vi "ABB SIgn All.vi"(11 "ImageFolder":path) -> ()   [LabVIEW 2017]
uses:
  ABB global.vi
panel:
  out "Signatures":T1(array[cluster])
  out "Please Sign":string
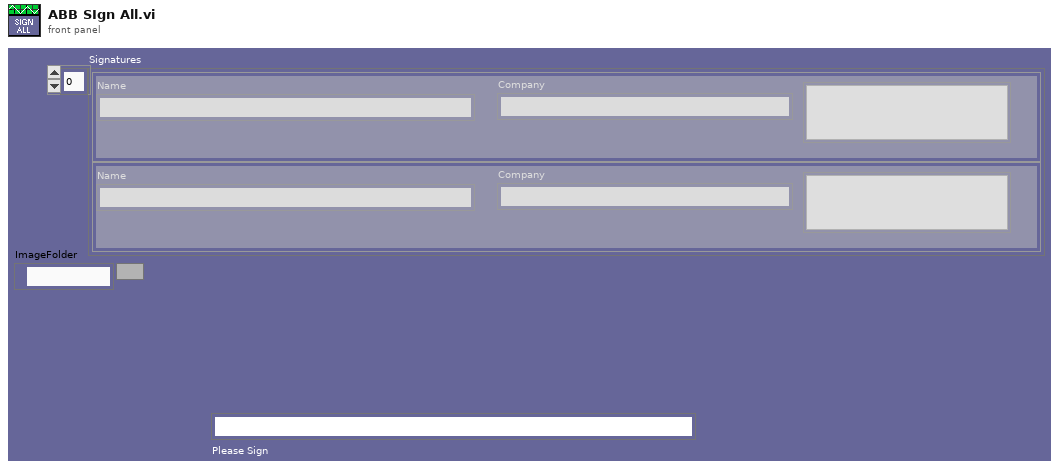
[diagram p1: front panel]
types:
  T1 = cluster{"Name":string, "Company":string, "new picture":picture}[]
  T2 = cluster{"String":string, "String":string, "new picture":picture}[]
  T3 = cluster{"String":string, "String":string, "Signature":picture}
  T4 = cluster{"String":string, "String":string, "Signature":picture}[]
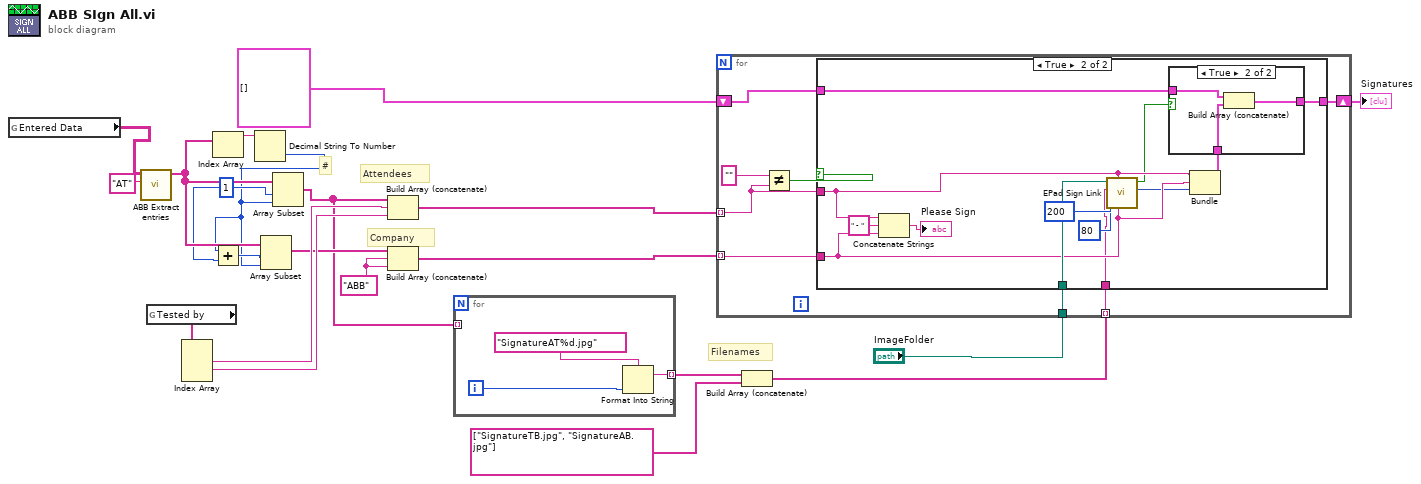
[diagram p0: block diagram]
diagram:
  w10 = "ABB"
  w18 = 1 ("index")
  # "Filenames"
  # "Company"
  # "Attendees"
  # "#"
  n1 = global read "ABB global.vi" "Entered Data"() -> (w15:string[][])
  n2 = call "ABB Extract entries.vi"("Entry ID"="AT", "Entry table in"=w15) -> ("Selected Entries"=w19:string[])  [unwired: 9 in]
  n3 = global read "ABB global.vi" "Tested by"() -> (w14:string[])
  n4 = Index Array(array=w14) -> (element #1=w13:string, element #2=w12:string)  [unwired: 3 in, 1 out]
  n5 = Index Array(array=w19) -> (element=w21:string)  [unwired: 1 in]
  n6 = Decimal String To Number(string=w21) -> (number=w16:i32)  [unwired: 2 in, 1 out]
  n7 = Add(x=w16, y=w18) -> (x+y=w17:i32)
  n8 = Array Subset(array=w19, index=w17, length=w16) -> (w11:string[])
  n9 = Array Subset(array=w19, index=w18, length=w16) -> (w2:string[])
  n10 = Build Array (concatenate)(w2, w13, w12) -> (w6:string[])
  n11 = Build Array (concatenate)(w11, w10, w10) -> (w9:string[])
  n12 = for {
    tunnel: [w22] -> w5 mode=indexing
    tunnel: w2 -> [_] mode=indexing
    i -> [w23]
    n13 = Format Into String(format string="SignatureAT%d.jpg" ("Filename"), w23) -> (resulting string=w22:string)  [unwired: 2 in, 1 out]
  }
  n14 = Build Array (concatenate)(w5, string[] ["SignatureTB.jpg", "SignatureAB.jpg"] ("element")) -> (w3:string[])
  n15 = for {
    tunnel: w6 -> [w30] mode=indexing
    tunnel: w9 -> [w32] mode=indexing
    tunnel: "ImageFolder" -> [w31]
    shift-right: [w27] -> w7
    shift-left: T2 [] -> [w26]
    tunnel: w3 -> [w25] mode=indexing
    n16 = Not Equal?(x="", y=w30) -> (x != y?=w28:bool)
    n17 = case shown="True" w28 {
      tunnel: w32 -> [_ w40]
      tunnel: w31 -> [_ w44]
      tunnel: w30 -> [_ w41]
      tunnel: [w33 w37] -> w27
      tunnel: w26 -> [w33 w36]
      tunnel: w25 -> [_ w34]
      frame False {
      }
      frame True {
        n18 = Concatenate Strings(w41, " - " ("string"), w40) -> (→"Please Sign":string)
        n19 = call "EPad Sign Link.vi"("OrgName"=w40, "Name"=w41, "e PadHeight"=80 ("nHeight"), "ePad Width"=200 ("nWidth"), "Filename"=w34, "Path"=w44) -> ("Signature"=w39:picture, "SignOK"=w35:bool)  [unwired: 4 in]
        n20 = Bundle("String"=w41, "String"=w40, "Signature"=w39) -> (w38:T3)  [unwired: 1 in]
        n21 = case shown="True" w35 {
          tunnel: w38 -> [_ w50]
          tunnel: [w47 w49] -> w37
          tunnel: w36 -> [w47 w48]
          frame False {
          }
          frame True {
            n22 = Build Array (concatenate)(w48, w50) -> (w49:T4)
          }
        }
      }
    }
  }
  "Signatures" <- w7
